vi "Merge.vi"() -> ()   [LabVIEW 2022 SP3]
panel:
  in  "Target folder":path
  out "file names path 1":string[](array[string])
  in  "pattern 2":string="*SFoc*"
  in  "pattern 1":string="*SumRing*"
  in  "right image":path
  in  "Ring":u16(ring)=1 items=["Split", "Merge"]
  out "file names path 2":string[](array[string])
  in  "left image":path
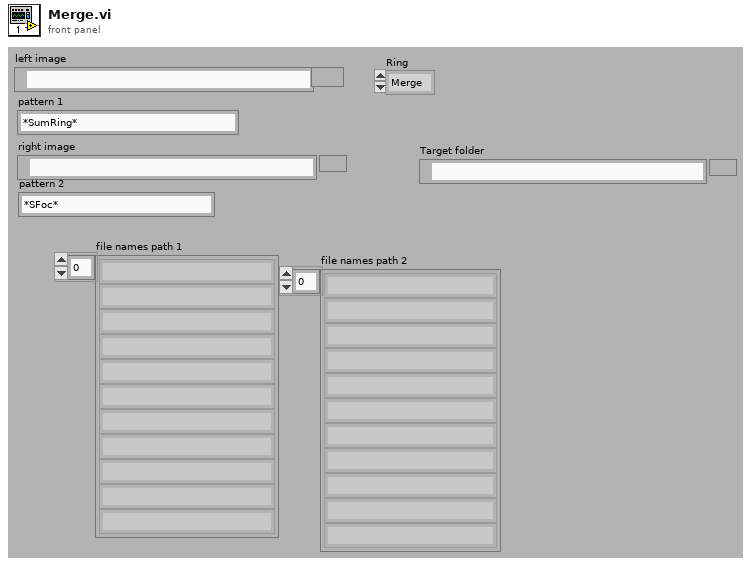
[diagram p1: front panel]
types:
  T1 = typedef "imagedata.ctl" = cluster{"image type":i32, "image depth":i32, "image":u8[], "mask":u8[], "colors":u32[], "Rectangle":cluster{"left":i16, "top":i16, "right":i16, "bottom":i16}}
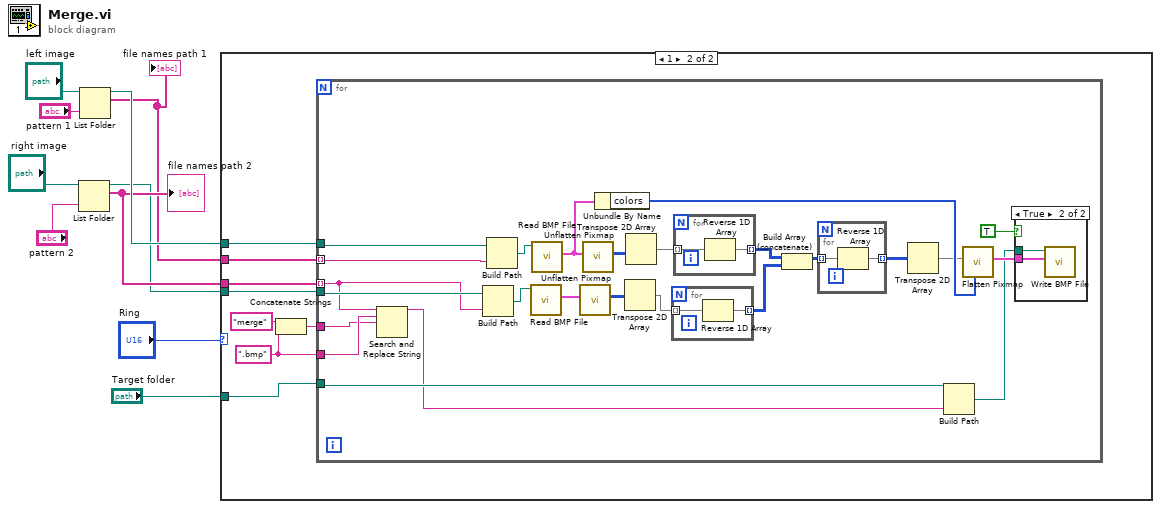
[diagram p0: block diagram]
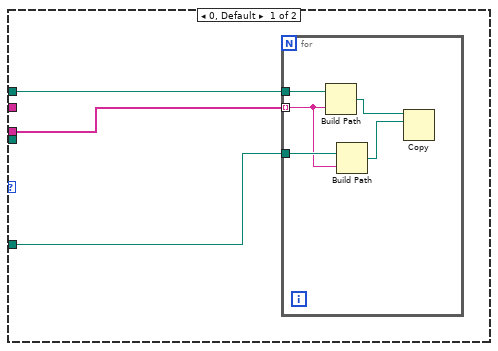
[diagram p2: hidden frame]
diagram:
  n1 = List Folder(path="right image", pattern="pattern 2") -> (path out=w5:path, filenames=w6:string[])  [unwired: 1 in, 3 out]
  "file names path 2" <- w6
  n2 = List Folder(path="left image", pattern="pattern 1") -> (path out=w10:path, filenames=w2:string[])  [unwired: 1 in, 3 out]
  "file names path 1" <- w2
  n3 = case shown="1" "Ring" {
    tunnel: w2 -> [_ w26]
    tunnel: w10 -> [w13 w25]
    tunnel: w6 -> [w12 w24]
    tunnel: w5 -> [_ w23]
    tunnel: "Target folder" -> [w11 w19]
    frame 0, Default {
      n4 = for {
        tunnel: w12 -> [w16] mode=indexing
        tunnel: w13 -> [w18]
        tunnel: w11 -> [w17]
        n5 = Build Path(base path=w18, name or relative path=w16) -> (appended path=w15:path)
        n6 = Build Path(base path=w17, name or relative path=w16) -> (appended path=w14:path)
        n7 = Copy(10:w14, 11:w15) -> ()  [unwired: 1 in, 5 out]
      }
    }
    frame 1 {
      w21 = ".bmp"
      n8 = Concatenate Strings("merge", w21) -> (w20:string)
      n9 = for {
        tunnel: w26 -> [w29] mode=indexing
        tunnel: w25 -> [w50]
        tunnel: w19 -> [w40]
        tunnel: w24 -> [w28] mode=indexing
        tunnel: w23 -> [w37]
        tunnel: w21 -> [w32]
        tunnel: w20 -> [w31]
        n10 = Search and Replace String(input string=w28, search string=w32, replace string=w31) -> (result string=w30:string)  [unwired: 1 in, 7 out]
        n11 = Build Path(base path=w37, name or relative path=w28) -> (appended path=w49:path)
        n12 = Build Path(base path=w50, name or relative path=w29) -> (appended path=w51:path)
        n13 = call <vilib>:"Read BMP File.vi"("path to BMP file"=w49) -> ("image data"=w47:T1)  [unwired: 1 in, 9 out]
        n14 = call <vilib>:"Read BMP File.vi"("path to BMP file"=w51) -> ("image data"=w48:T1)  [unwired: 1 in, 9 out]
        n15 = call <vilib>:"Unflatten Pixmap.vi"("image data"=w47) -> ("8-bit pixmap"=w41:u8[][])  [unwired: 10 out]
        n16 = call <vilib>:"Unflatten Pixmap.vi"("image data"=w48) -> ("8-bit pixmap"=w42:u8[][])  [unwired: 10 out]
        n17 = Unbundle By Name(w48) -> ("colors"=w45:u32[])
        n18 = Transpose 2D Array(2D array=w41) -> (transposed array=w34:u8[][])
        n19 = Transpose 2D Array(2D array=w42) -> (transposed array=w43:u8[][])
        n20 = for {
          tunnel: w34 -> [w55] mode=indexing
          tunnel: [w54] -> w33 mode=indexing
          n21 = Reverse 1D Array(array=w55) -> (reversed array=w54:u8[])
        }
        n22 = for {
          tunnel: w43 -> [w59] mode=indexing
          tunnel: [w58] -> w36 mode=indexing
          n23 = Reverse 1D Array(array=w59) -> (reversed array=w58:u8[])
        }
        n24 = Build Array (concatenate)(w36, w33) -> (w39:u8[][])
        n25 = for {
          tunnel: [w57] -> w38 mode=indexing
          tunnel: w39 -> [w56] mode=indexing
          n26 = Reverse 1D Array(array=w56) -> (reversed array=w57:u8[])
        }
        n27 = Transpose 2D Array(2D array=w38) -> (transposed array=w35:u8[][])
        n28 = Build Path(base path=w40, name or relative path=w30) -> (appended path=w44:path)
        n29 = call <vilib>:"Flatten Pixmap.vi"("colors"=w45, "8-bit pixmap"=w35) -> ("image data"=w46:T1)  [unwired: 4 in, 5 out]
        n30 = case shown="True" TRUE {
          tunnel: w46 -> [_ w53]
          tunnel: w44 -> [_ w52]
          frame False {
          }
          frame True {
            n31 = call <vilib>:"Write BMP File.vi"("image data"=w53, "path to BMP file"=w52) -> ()  [unwired: 1 in, 9 out]
          }
        }
      }
    }
  }
